vi "Set_R_C.vi"(10 "Value":i32, 11 "Value 2":i32) -> (2 "簇":cluster{"Value":i32, "Value":i32}, 3 "数值":i32)   [LabVIEW 2018]
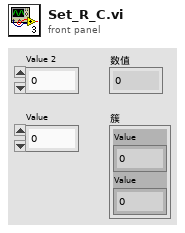
[diagram p1: front panel]
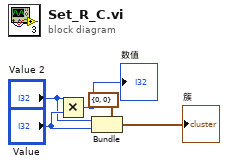
[diagram p0: block diagram]
diagram:
  n1 = Multiply(x="Value 2", y="Value") -> (x*y=→"数值":i32)
  n2 = Bundle(cluster=cluster{"Value":i32, "Value":i32} {"Value"=0, "Value"=0} ("簇"), "Value"="Value 2", "Value"="Value") -> (→"簇":cluster{"Value":i32, "Value":i32})
